vi "Client LabVIEW.vi"() -> ()   [LabVIEW 2014]
panel:
  out "Missatge del servidor":string
  in  "Missatge del client":string
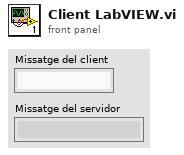
[diagram p1: front panel]
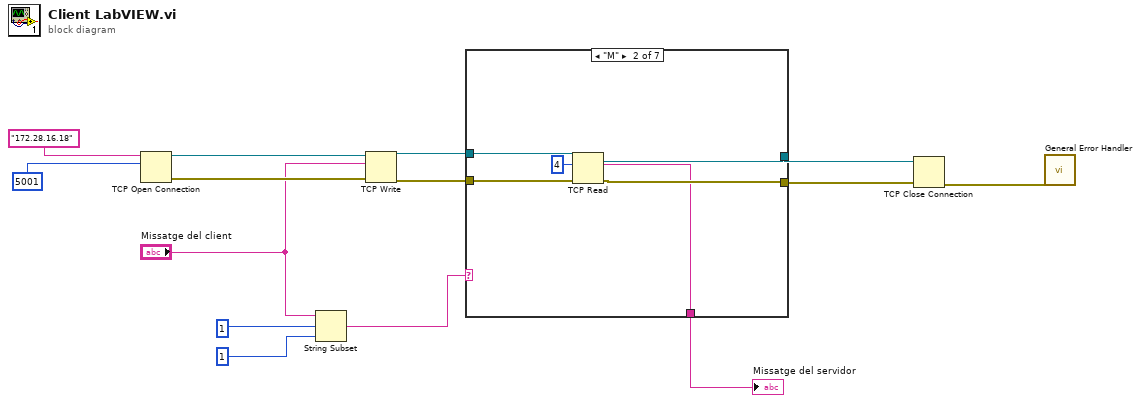
[diagram p0: block diagram]
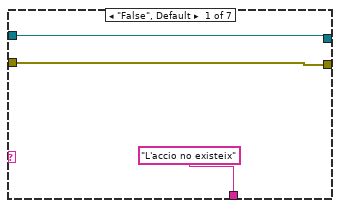
[diagram p2: hidden frame]
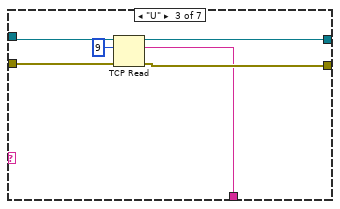
[diagram p3: hidden frame]
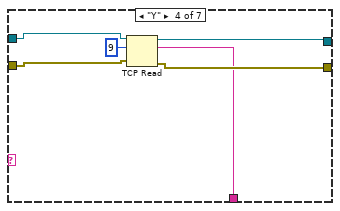
[diagram p4: hidden frame]
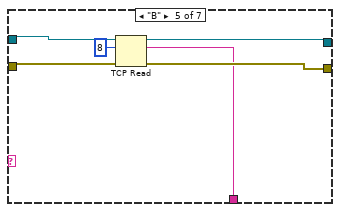
[diagram p5: hidden frame]
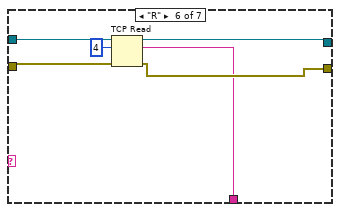
[diagram p6: hidden frame]
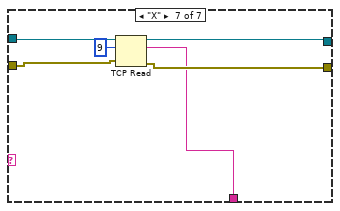
[diagram p7: hidden frame]
diagram:
  n1 = TCP Open Connection(address="172.28.16.18", remote port or service name=u16 5001) -> (connection ID=w12:refnum<k5>, error out=w11:errorcluster)  [unwired: 3 in]
  n2 = String Subset(string="Missatge del client", offset (0)=1, length (rest)=1 ("length (rest)")) -> (substring=w8:string)
  n3 = TCP Write(connection ID=w12, data in="Missatge del client", error in (no error)=w11) -> (connection ID out=w6:refnum<k5>, error out=w5:errorcluster)  [unwired: 1 in, 1 out]
  n4 = case shown="\"M\"" w8 {
    tunnel: w6 -> [w17 w22 w28 w34 w40 w46 w52]
    tunnel: w5 -> [w16 w21 w27 w33 w39 w45 w51]
    tunnel: [w17 w20 w25 w32 w38 w44 w50] -> w4
    tunnel: [w16 w19 w26 w31 w37 w43 w49] -> w3
    tunnel: ["L'accio no existeix" ("data out") w18 w24 w30 w36 w42 w48] -> w2
    frame "False", Default {
    }
    frame "M" {
      n5 = TCP Read(connection ID=w22, bytes to read=4, error in (no error)=w21) -> (connection ID out=w20:refnum<k5>, data out=w18:string, error out=w19:errorcluster)  [unwired: 2 in]
    }
    frame "U" {
      n6 = TCP Read(connection ID=w28, bytes to read=9, error in (no error)=w27) -> (connection ID out=w25:refnum<k5>, data out=w24:string, error out=w26:errorcluster)  [unwired: 2 in]
    }
    frame "Y" {
      n7 = TCP Read(connection ID=w34, bytes to read=9, error in (no error)=w33) -> (connection ID out=w32:refnum<k5>, data out=w30:string, error out=w31:errorcluster)  [unwired: 2 in]
    }
    frame "B" {
      n8 = TCP Read(connection ID=w40, bytes to read=8, error in (no error)=w39) -> (connection ID out=w38:refnum<k5>, data out=w36:string, error out=w37:errorcluster)  [unwired: 2 in]
    }
    frame "R" {
      n9 = TCP Read(connection ID=w46, bytes to read=4, error in (no error)=w45) -> (connection ID out=w44:refnum<k5>, data out=w42:string, error out=w43:errorcluster)  [unwired: 2 in]
    }
    frame "X" {
      n10 = TCP Read(connection ID=w52, bytes to read=9, error in (no error)=w51) -> (connection ID out=w50:refnum<k5>, data out=w48:string, error out=w49:errorcluster)  [unwired: 2 in]
    }
  }
  "Missatge del servidor" <- w2
  n11 = TCP Close Connection(connection ID=w4, error in (no error)=w3) -> (error out=w14:errorcluster)  [unwired: 1 in, 1 out]
  n12 = call <vilib>:"General Error Handler.vi"("error in (no error)"=w14) -> ()  [unwired: 10 in, 5 out]
